vi "Server monitor.vi"() -> ()   [LabVIEW 2010]
uses:
  DAQ configuration/channel identifier.ctl
panel:
  out "error out":errorcluster
  out "Range Error":bool
  out "arbitrary time (s)":dbl format="%.2f"
  in  "Port":T1
  in  "millisecond multiple":u32=1000
  in  "stop":bool
  out "voltage data":sgl format="%.5f"
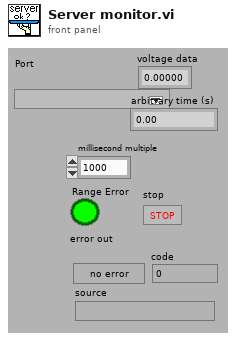
[diagram p1: front panel]
types:
  T1 = typedef "channel identifier.ctl" = u16
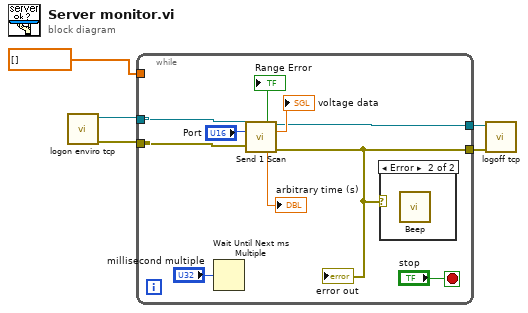
[diagram p0: block diagram]
diagram:
  n1 = call "logon enviro tcp.vi"() -> ("error out"=w3:errorcluster, "connection ID"=w4:refnum<k5>)  [unwired: 9 in, 1 out]
  n2 = while {
    tunnel: sgl[] [] ("History Data") -> [_]
    tunnel: [w10] -> w2
    tunnel: w3 -> [w14]
    tunnel: w4 -> [w15]
    tunnel: [w6] -> w5
    stop <- "stop" stop-if-true
    n3 = Wait Until Next ms Multiple(millisecond multiple="millisecond multiple") -> ()  [unwired: 1 out]
    n4 = call "Send 1 Scan.vi"("Connection ID in"=w15, "Port"="Port", "error in (no error)"=w14) -> ("Out of Range"=→"Range Error":bool, "Connection ID out"=w10:refnum<k5>, "voltage data"=→"voltage data":sgl, "Time"=→"arbitrary time (s)":dbl, "error out"=w6:errorcluster)  [unwired: 5 in, 3 out]
    "error out" <- w6
    n5 = case shown="Error" w6 {
      frame No Error {
      }
      frame Error {
        n6 = call <vilib>:"Beep.vi"() -> ()  [unwired: 12 in]
      }
    }
  }
  n7 = call "logoff tcp.vi"("error in (no error)"=w5, "Connection ID"=w2) -> ()  [unwired: 8 in, 2 out]
